vi "GT Buf Enable Do Bit Pulse.vi"(0 "cardNum":i16, 1 "highLevelTime":u16, 2 "pulseNum":i32, 3 "fifo":i16, 5 "crd":i16, 7 "doType":i16, 9 "doIndex":i16, 11 "error in (no error)":errorcluster caption="错误输入（无错误）", 12 "lowLevelTime":u16, 13 "firstLevel":i16) -> (4 "function return":i16, 15 "error out":errorcluster caption="错误输出")   [LabVIEW 2020, in "gts.lvlib"]
doc: "GT_API GT_BufEnableDoBitPulse(short cardNum,short crd,short doType,short doIndex,unsigned short highLevelTime,unsigned short lowLevelTime,long pulseNum,short firstLevel,short fifo=0);"
uses:
  gts.lvlib
  dll/32bit/multi_card/gts.dll
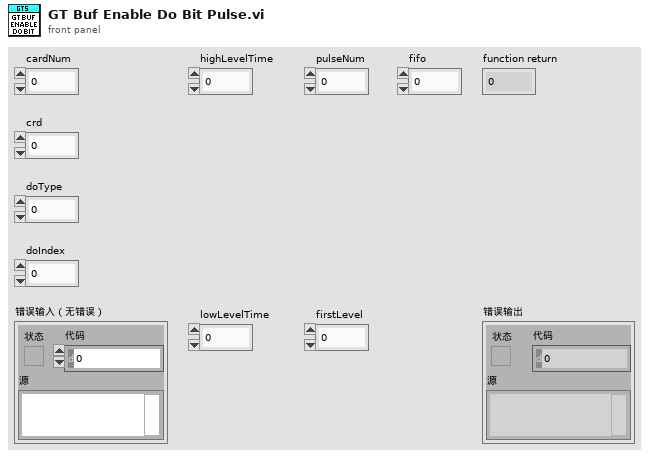
[diagram p1: front panel]
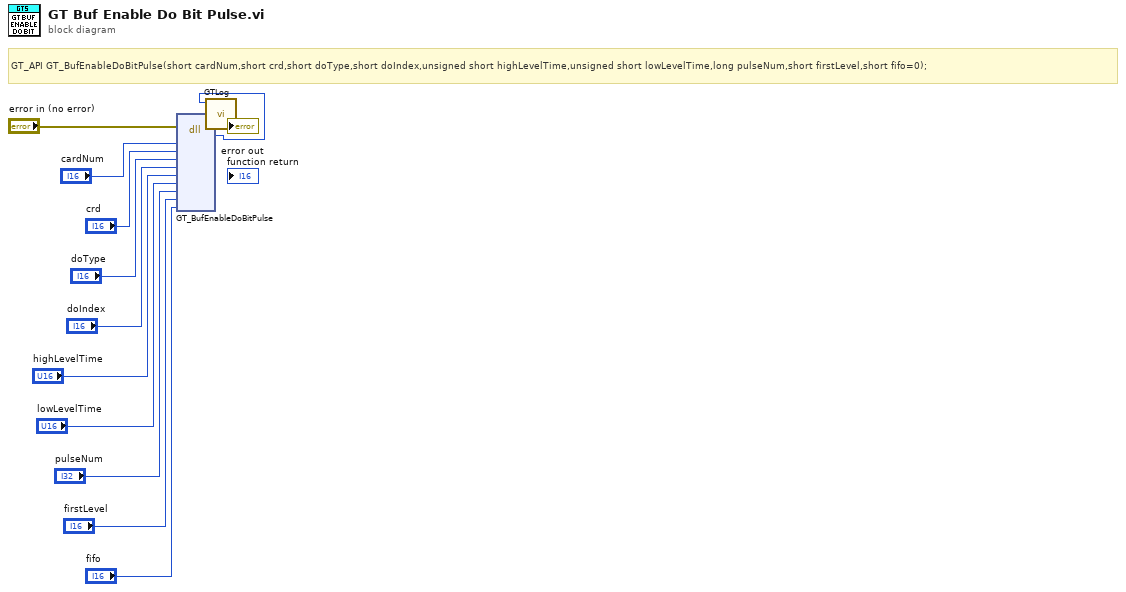
[diagram p0: block diagram]
diagram:
  # "GT_API GT_BufEnableDoBitPulse(short cardNum,short crd,short doType,short doIndex,unsigned short highLevelTime,unsigned short lowLevelTime,long pulseNum,short firstLevel,short fifo=0);"
  n1 = dll-call lib="C:/1228/dll/32bit/multi_card/gts.dll" fn="GT_BufEnableDoBitPulse"(error in="error in (no error)", "cardNum"="cardNum", "crd"="crd", "doType"="doType", "doIndex"="doIndex", "highLevelTime"="highLevelTime", "lowLevelTime"="lowLevelTime", "pulseNum"="pulseNum", "firstLevel"="firstLevel", "fifo"="fifo") -> (error out=w3:errorcluster, w1:i16)  [unwired: 11 in, 1 out]
  n2 = call "GTLog.vi"("error in (no error)"=w3, "Numeric"=w1) -> ("error out"=→"error out":errorcluster)  [unwired: 9 in]
